vi "Wait For Packet.vi"(7 "Timeout (100 ms)":i32=100, 8 "Error In":errorcluster, 11 "LINX Device Config":T1={"Interface"=enum."TCP", "COM Port"="COM5", "TCP Configuration"={"IP Address"="10.2.106.213", "Port"=6921}, "Device Family"=1, "Device ID"=1, "Device Name"="chipKIT uC32", "TCP Ref"=refnum, "Channels"={"DI"=[], "DO"=[], "AI"=[], "AO"=[], "PWM"=[], "QE"=[], "UART"=[], "I2C 2"=[], "SPI"=[], "CAN"=[], "Servo"=[], "AI Ref (V)"=0.0, "AI Resolution (Bits)"=0, "AO Ref (V)"=0.0, "AO Resolution (Bits)"=0}}) -> (0 "Error Out":errorcluster, 2 "Packet":u8[](array[numeric])=[255, 6, 0, 66, 0, 71], 3 "LINX Device Config":T1={"Interface"=enum."TCP", "COM Port"="COM5", "TCP Configuration"={"IP Address"="10.2.106.213", "Port"=6921}, "Device Family"=1, "Device ID"=1, "Device Name"="chipKIT uC32", "TCP Ref"=refnum, "Channels"={"DI"=[], "DO"=[], "AI"=[], "AO"=[], "PWM"=[], "QE"=[], "UART"=[], "I2C 2"=[], "SPI"=[], "CAN"=[], "Servo"=[], "AI Ref (V)"=0.0, "AI Resolution (Bits)"=0, "AO Ref (V)"=0.0, "AO Resolution (Bits)"=0}})   [LabVIEW 2020, in "LMH-LINX.lvlib" / "Device.lvlib"]
doc: "Wait until a LINX return packet is received or a timout occurs. If a valid packet is recieved this VI will return that packet otherwise this VI returns and empty packet and generates an error."
uses:
  Device.lvlib
  Type Defs/LINX Device Config.ctl
  Type Defs/Interface.ctl
  Type Defs/TCP Config.ctl
  Type Defs/Channels.ctl
  Type Defs/Error Type.ctl
  LMH-LINX.lvlib
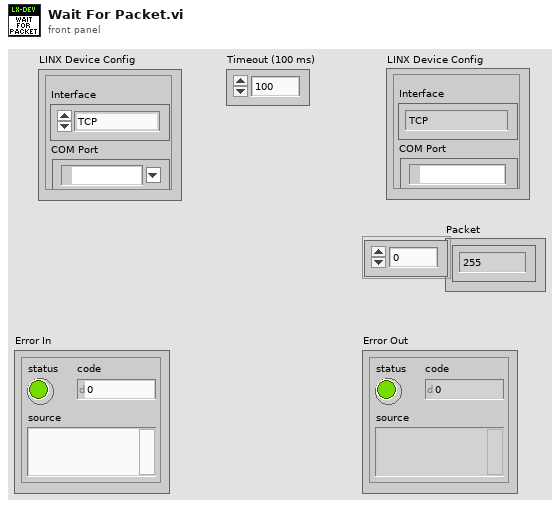
[diagram p1: front panel]
types:
  T1 = typedef "LMH-LINX.lvlib/Device.lvlib/LINX Device Config.ctl" = cluster{"Interface":T2, "COM Port":refnum<visa-resource-name>, "TCP Configuration":T3, "Device Family":u8, "Device ID":u8, "Device Name":string, "TCP Ref":refnum<k5>, "Channels":T4}
  T2 = typedef "LMH-LINX.lvlib/Interface.ctl" = enum16{"Serial", "TCP"}
  T3 = typedef "LMH-LINX.lvlib/Device.lvlib/TCP Config.ctl" = cluster{"IP Address":string, "Port":u16}
  T4 = typedef "LMH-LINX.lvlib/Channels.ctl" = cluster{"DI":u8[], "DO":u8[], "AI":u8[], "AO":u8[], "PWM":u8[], "QE":u8[], "UART":u8[], "I2C 2":u8[], "SPI":u8[], "CAN":u8[], "Servo":u8[], "AI Ref (V)":dbl, "AI Resolution (Bits)":u8, "AO Ref (V)":dbl, "AO Resolution (Bits)":u8}
  T5 = typedef "LMH-LINX.lvlib/Error Type.ctl" = enum16{"Unknown", "Timeout", "Corrupt Return Packet", "Unable To Connect", "Command Not Supported", "Channel DNE", "Invalid COM Config", "Firmware Version Mismatch", "myRIO Support", "CMD Specific Error", "Local IO Not Supported"}
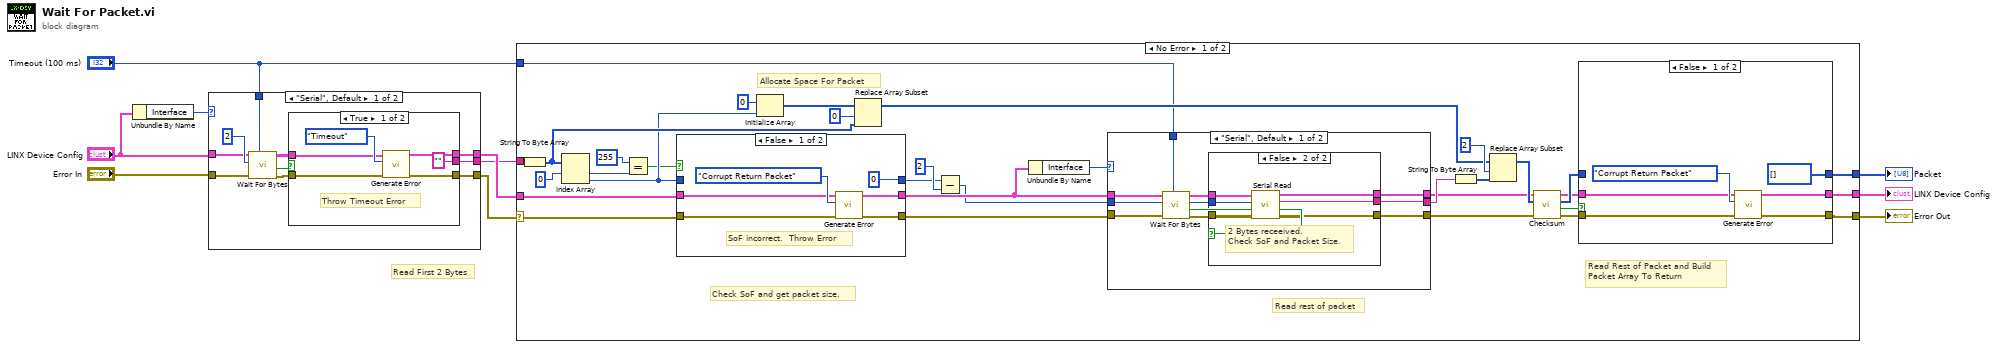
[diagram p0: block diagram]
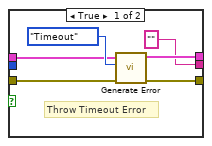
[diagram p4: hidden frame]
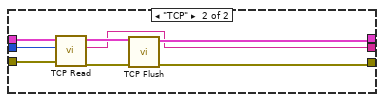
[diagram p5: hidden frame]
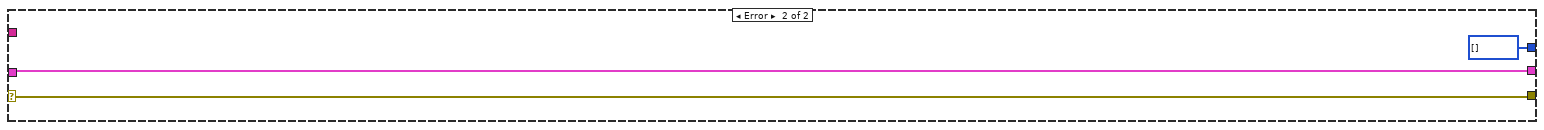
[diagram p6: hidden frame]
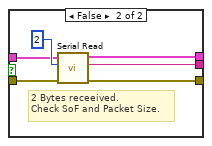
[diagram p7: hidden frame]
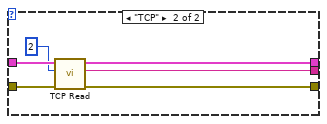
[diagram p8: hidden frame]
diagram:
  # "Read First 2 Bytes"
  n1 = Unbundle By Name("LINX Device Config") -> ("Interface"=w10:T2)
  n2 = case shown="\"Serial\", Default" w10 {
    tunnel: "Error In" -> [w19 w37]
    tunnel: "LINX Device Config" -> [w18 w38]
    tunnel: [w14 w36] -> w7
    tunnel: [w13 w35] -> w1
    tunnel: [w12 w33] -> w6
    tunnel: "Timeout (100 ms)" -> [w11 _]
    frame "Serial", Default {
      n3 = call "Wait For Bytes.vi"("Timeout (100 ms)"=w11, "Error In"=w19, "Num Bytes"=u32 2, "LINX Device Config"=w18) -> ("Error Out"=w15:errorcluster, "Timeout"=w17:bool, "LINX Device Config"=w16:T1)  [unwired: 4 in, 1 out]
      n4 = case shown="True" w17 {
        tunnel: w16 -> [w25 w31]
        tunnel: w15 -> [w24 w30]
        tunnel: [w23 w29] -> w14
        tunnel: [w22 w28] -> w13
        tunnel: ["" ("Data") w27] -> w12
        frame True {
          # "Throw Timeout Error"
          n5 = call "Generate Error.vi"("Error In"=w24, "Error Type"=Error_Type."Timeout", "LINX Device Config"=w25) -> ("Error Out"=w22:errorcluster, "Dup LINX Device Config"=w23:T1)  [unwired: 7 in]
        }
        frame False {
          # "2 Bytes receeived.  \nCheck SoF and Packet Size."
          n6 = call "Serial Read.vi"("Error In"=w30, "Bytes To Read"=u32 2 ("byte count"), "LINX Device Config"=w31) -> ("Error Out"=w28:errorcluster, "Data"=w27:string, "LINX Device Config"=w29:T1)  [unwired: 6 in]
        }
      }
    }
    frame "TCP" {
      n7 = call "TCP Read.vi"("Error In"=w37, "Bytes To Read"=u32 2 ("Num Bytes"), "LINX Device Config"=w38) -> ("Error Out"=w35:errorcluster, "Data"=w33:string, "LINX Device Config"=w36:T1)  [unwired: 6 in]
    }
  }
  n8 = case shown="No Error" w1 {
    selector: w1 -> [w39 w123]
    tunnel: w7 -> [w71 w121]
    tunnel: w6 -> [w70 _]
    tunnel: [w55 w123] -> w5
    tunnel: [w54 w121] -> w4
    tunnel: [w53 u8[] [] ("Packet")] -> w3
    tunnel: "Timeout (100 ms)" -> [w52 _]
    frame No Error {
      # "Allocate Space For Packet"
      # "Read Rest of Packet and Build\nPacket Array To Return"
      # "Read rest of packet"
      # "Check SoF and get packet size."
      n9 = String To Byte Array(string=w70) -> (unsigned byte array=w48:u8[])
      n10 = Index Array(array=w48, index #1=0 ("index")) -> (element #1=w41:u8, element #2=w44:u8)  [unwired: 1 in]
      n11 = Equal?(x=u8 255, y=w41) -> (x = y?=w43:bool)
      n12 = case shown="False" w43 {
        tunnel: w44 -> [_ w78]
        tunnel: w39 -> [w77 w80]
        tunnel: [w76 w80] -> w67
        tunnel: [w73 w79] -> w69
        tunnel: w71 -> [w74 w79]
        tunnel: [u8 0 w78] -> w49
        frame False {
          # "SoF incorrect.  Throw Error"
          n13 = call "Generate Error.vi"("Error In"=w77, "Error Type"=Error_Type."Corrupt Return Packet", "LINX Device Config"=w74) -> ("Error Out"=w76:errorcluster, "Dup LINX Device Config"=w73:T1)  [unwired: 7 in]
        }
        frame True {
          # "SoF Correct.  Continue Reading Packet"
        }
      }
      n14 = Initialize Array(u8 0 ("element"), w44) -> (w46:u8[])
      n15 = Replace Array Subset(array=w46, new element=w48, index=0) -> (w56:u8[])
      n16 = Subtract(x=w49, y=u8 2) -> (x-y=w51:u8)
      n17 = Unbundle By Name(w69) -> ("Interface"=w68:T2)
      n18 = case shown="\"Serial\", Default" w68 {
        tunnel: w67 -> [w100 w119]
        tunnel: w69 -> [w99 w120]
        tunnel: [w95 w116] -> w57
        tunnel: [w94 w114] -> w59
        tunnel: [w93 w113] -> w58
        tunnel: w52 -> [w92 _]
        tunnel: w51 -> [w91 w118]
        frame "Serial", Default {
          n19 = call "Wait For Bytes.vi"("Timeout (100 ms)"=w92, "Error In"=w100, "Num Bytes"=w91, "LINX Device Config"=w99) -> ("Error Out"=w96:errorcluster, "Timeout"=w98:bool, "Num Bytes"=w90:u32, "LINX Device Config"=w97:T1)  [unwired: 4 in]
          n20 = case shown="False" w98 {
            tunnel: w97 -> [w105 w112]
            tunnel: w96 -> [w104 w111]
            tunnel: [w103 w110] -> w95
            tunnel: [w102 w109] -> w94
            tunnel: ["" ("Data") w108] -> w93
            tunnel: w90 -> [_ w107]
            frame True {
              # "Throw Timeout Error"
              n21 = call "Generate Error.vi"("Error In"=w104, "Error Type"=Error_Type."Timeout", "LINX Device Config"=w105) -> ("Error Out"=w102:errorcluster, "Dup LINX Device Config"=w103:T1)  [unwired: 7 in]
            }
            frame False {
              # "2 Bytes receeived.  \nCheck SoF and Packet Size."
              n22 = call "Serial Read.vi"("Error In"=w111, "Bytes To Read"=w107, "LINX Device Config"=w112) -> ("Error Out"=w109:errorcluster, "Data"=w108:string, "LINX Device Config"=w110:T1)  [unwired: 6 in]
            }
          }
        }
        frame "TCP" {
          n23 = call "TCP Read.vi"("Error In"=w119, "Bytes To Read"=w118, "LINX Device Config"=w120) -> ("Error Out"=w115:errorcluster, "Data"=w113:string, "LINX Device Config"=w117:T1)  [unwired: 6 in]
          n24 = call "TCP Flush.vi"("Error In"=w115, "LINX Device Config"=w117) -> ("Error Out"=w114:errorcluster, "LINX Device Config"=w116:T1)  [unwired: 7 in, 1 out]
        }
      }
      n25 = String To Byte Array(string=w58) -> (unsigned byte array=w61:u8[])
      n26 = Replace Array Subset(array=w56, new element=w61, index=2) -> (w62:u8[])
      n27 = call "Checksum.vi"("Error In"=w59, "Packet"=w62, "LINX Device Config"=w57) -> ("Error Out"=w64:errorcluster, "Checksum Pass?"=w65:bool, "Packet"=w66:u8[], "LINX Device Config"=w63:T1)  [unwired: 5 in]
      n28 = case shown="False" w65 {
        tunnel: [w86 w89] -> w55
        tunnel: w64 -> [w85 w89]
        tunnel: [w82 w88] -> w54
        tunnel: w63 -> [w83 w88]
        tunnel: w66 -> [_ w87]
        tunnel: [u8[] [] w87] -> w53
        frame False {
          n29 = call "Generate Error.vi"("Error In"=w85, "Error Type"=Error_Type."Corrupt Return Packet", "LINX Device Config"=w83) -> ("Error Out"=w86:errorcluster, "Dup LINX Device Config"=w82:T1)  [unwired: 7 in]
        }
        frame True {
          # "Checksum Passed\nReturn Valid Packet"
        }
      }
    }
    frame Error {
    }
  }
  "Error Out" <- w5
  "Packet" <- w3
  "LINX Device Config" <- w4
